vi "DeviceOn.vi"(8 "error in (no error)":errorcluster, 11 "ChromaAcLoad in":refnum<class "ChromaAcLoad.lvclass">) -> (0 "error out":errorcluster, 3 "ChromaAcLoad out":refnum<class "ChromaAcLoad.lvclass">)   [LabVIEW 2018, in "AcPwrPlugins.lvlib" / "ChromaAcLoad.lvclass"]
doc: "This VI enables the output."
uses:
  ChromaAcLoad.lvclass
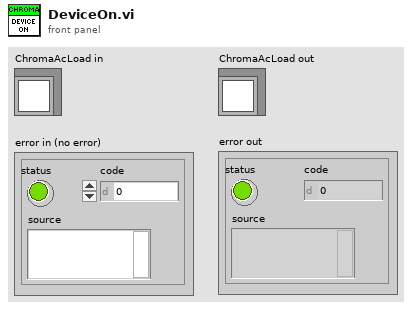
[diagram p1: front panel]
types:
  T1 = cluster{"Handle":string, "Name":string, "Phase Select":i32, "Instrument Options":string, "id query (T)":bool, "reset device (T)":bool, "Load Short Circuited":bool, "Line Synchronization":bool, "Load Current (A/Arms)":dbl, "Load Voltage (V/Vrms)":dbl, "Load Power (W)":dbl, "Load Resistance (Ohms)":dbl, "Load Current Peak Limit (A)":dbl, "Load Current Limit (A/Arms)":dbl, "Load Power Limit (W)":dbl, "Synch Frequency (Hz)":dbl, "Priority":enum16{"CF Only", "PF Only", "Both (CF)", "Both (PF)"}, "Crest Factor":dbl, "Power Factor":dbl, "Slew Rate":cluster{"Rise Slew Rate (A/ms)":i32, "Fall Slew Rate (A/ms)":i32}, "LC/RLC Mode":cluster{"Capacitance (uF)":i32, "Inductance (uH)":i32, "Series Resistance (Ohm)":dbl, "Parallel Resistance (Ohm)":dbl}, "Timing":cluster{"TimingOn":enum16{""}, "Hours":u32, "Minutes":u32, "Seconds":dbl, "CutoffVoltage":dbl}, "Connected":bool}[]
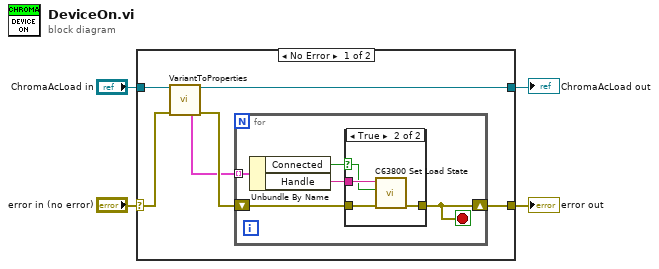
[diagram p0: block diagram]
diagram:
  n1 = case shown="No Error" "error in (no error)" {
    selector: "error in (no error)" -> [w7 w22]
    tunnel: [w10 w22] -> w1
    tunnel: [w9 w21] -> w4
    tunnel: "ChromaAcLoad in" -> [w8 w21]
    frame No Error {
      n2 = call "VariantToProperties.vi"("ChromaAcLoad"=w8, "error in (no error)"=w7) -> ("ChromaAcLoad"=w9:refnum<class "ChromaAcLoad.lvclass">, "Phases"=w5:T1, "error out"=w6:errorcluster)  [unwired: 7 in, 4 out]
      n3 = for {
        tunnel: w5 -> [w15] mode=indexing
        shift-right: [w12] -> w10
        shift-left: w6 -> [w14]
        stop <- w12 stop-if-true
        n4 = Unbundle By Name(w15) -> ("Connected"=w11:bool, "Handle"=w13:string)
        n5 = case shown="True" w11 {
          selector: w11 -> [_ w17]
          tunnel: w14 -> [w16 w20]
          tunnel: w13 -> [_ w19]
          tunnel: [w16 w18] -> w12
          frame False {
          }
          frame True {
            n6 = call <instrlib>:"C63800 Set Load State.vi"("error in (no error)"=w20, "Load State"=w17, "Instrument Handle"=w19) -> ("error out"=w18:errorcluster)  [unwired: 7 in, 1 out]
          }
        }
      }
    }
    frame Error {
    }
  }
  "error out" <- w1
  "ChromaAcLoad out" <- w4
